vi "Measurement Logic.vi"() -> ()   [LabVIEW 2021, in "Multi-Channel Output Voltage Accuracy_PMIC.lvlib"]
uses:
  Multi-Channel Output Voltage Accuracy_PMIC.lvlib
  <instrlib>/niDCPower/nidcpower.llb/niDCPower Sense.ctl
  <instrlib>/niDCPower/nidcpower.llb/niDCPower Source Mode.ctl
  <instrlib>/niDCPower/nidcpower.llb/niDCPower Get Channel Name From String.vi
  <instrlib>/niDCPower/nidcpower.llb/niDCPower Wait For Event - Event.ctl
  Measurement Results.ctl
  <instrlib>/niDCPower/nidcpower.llb/niDCPower Configure Digital Edge Source Trigger.vi
  <instrlib>/niDCPower/nidcpower.llb/niDCPower Configure Digital Edge Measure Trigger.vi
  Measurement Configuration.ctl
  <vilib>/Plug-In SDKs/Measurements/Measure Call Context/Measure Call Context.lvclass
panel:
  out "measure call context out":refnum<class "Measure Call Context.lvclass">
  in  "measure call context in":refnum<class "Measure Call Context.lvclass">
  out "measurement results":T1
  in  "measurement configuration":T2={"Mode of operation"=enum."Perform measurement", "DUT setup time"=1.0, "Aperture time"=0.005, "Measurement time"=1.0, "Source resource name"="", "Source voltage level"=6.0, "Source current limit"=10.0, "Load resource names"=[], "Output channel alias"=[], "Load current levels"=[], "Load voltage limit ranges"=[], "Nominal output voltages"=[]} {"Measurement time" format="%.3p"}
  out "error out":errorcluster
  in  "error in":errorcluster
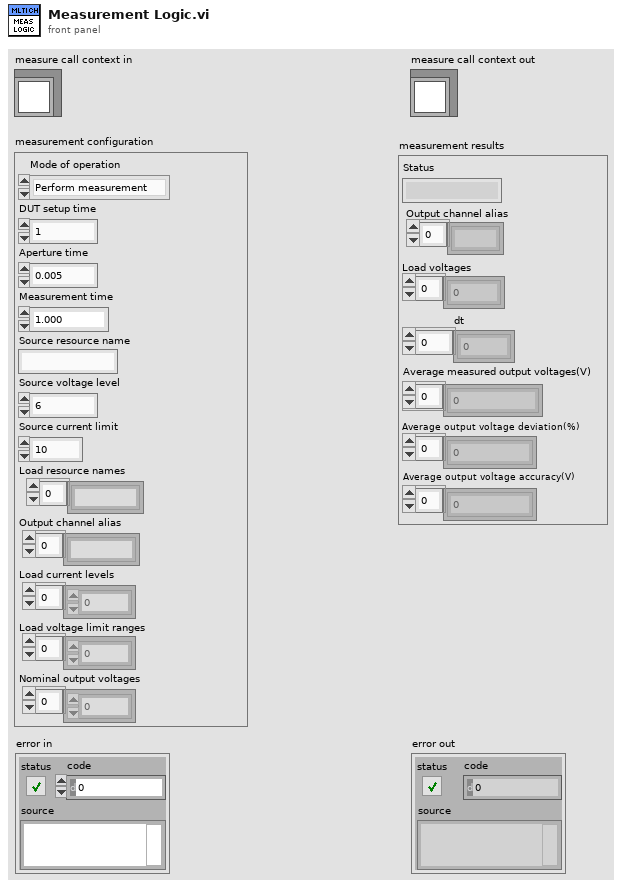
[diagram p1: front panel]
types:
  T1 = typedef "Multi-Channel Output Voltage Accuracy_PMIC.lvlib/Measurement Results.ctl" = cluster{"Status":string, "Output channel alias":string[], "Load voltages":dbl[], "dt":dbl[], "Average measured output voltages(V)":dbl[], "Average output voltage deviation(%)":dbl[], "Average output voltage accuracy(V)":dbl[]}
  T2 = typedef "Multi-Channel Output Voltage Accuracy_PMIC.lvlib/Measurement Configuration.ctl" = cluster{"Mode of operation":enum32{"Power on the DUT", "Perform measurement", "Power off the DUT"}, "DUT setup time":dbl, "Aperture time":dbl, "Measurement time":dbl, "Source resource name":string, "Source voltage level":dbl, "Source current limit":dbl, "Load resource names":string[], "Output channel alias":string[], "Load current levels":dbl[], "Load voltage limit ranges":dbl[], "Nominal output voltages":dbl[]}
  T3 = enum32{"Power on the DUT", "Perform measurement", "Power off the DUT"}
  T4 = typedef "niDCPower Wait For Event - Event.ctl" = i32
  T5 = typedef "niDCPower Source Mode.ctl" = i32
  T6 = typedef "niDCPower Sense.ctl" = i32
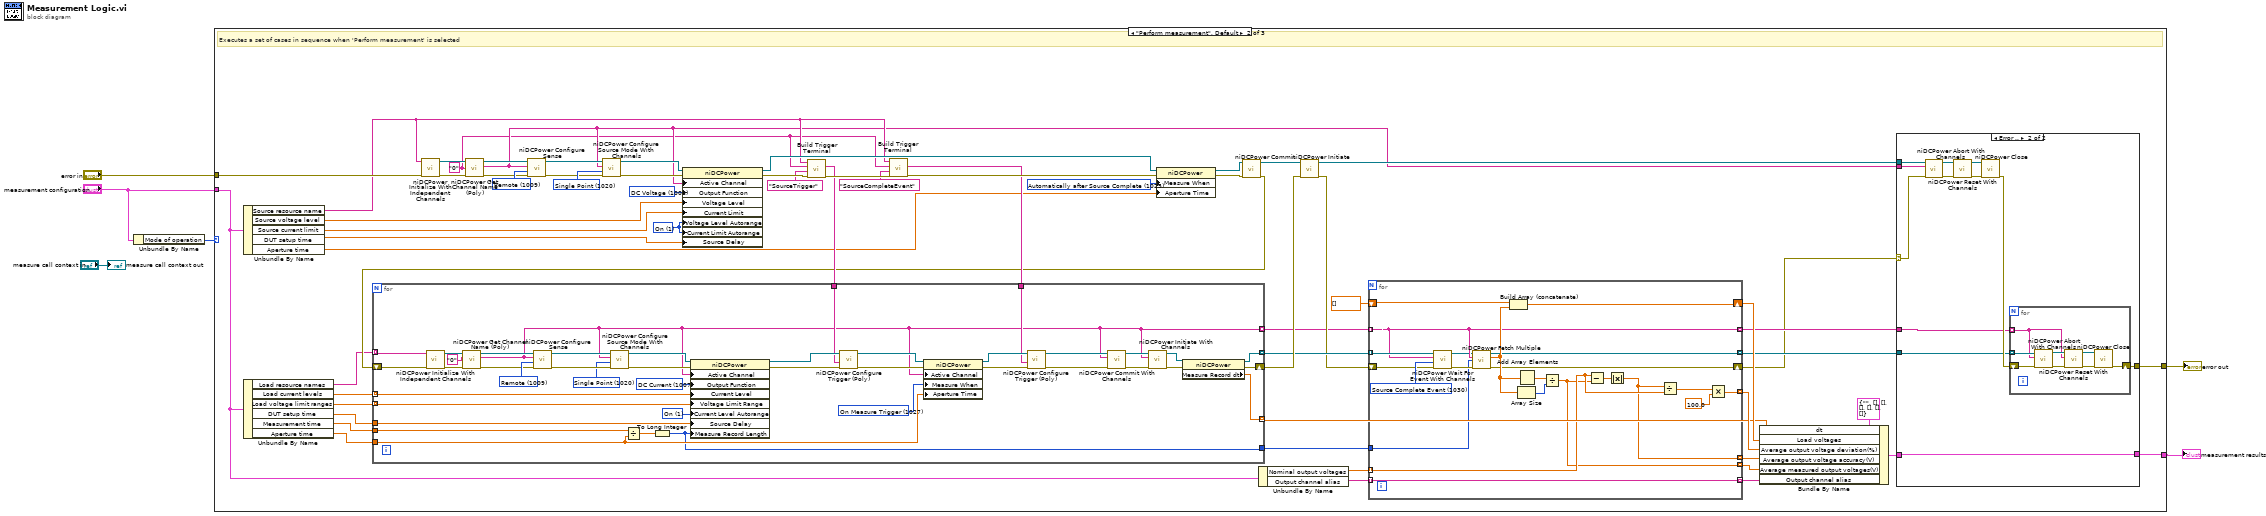
[diagram p0: block diagram]
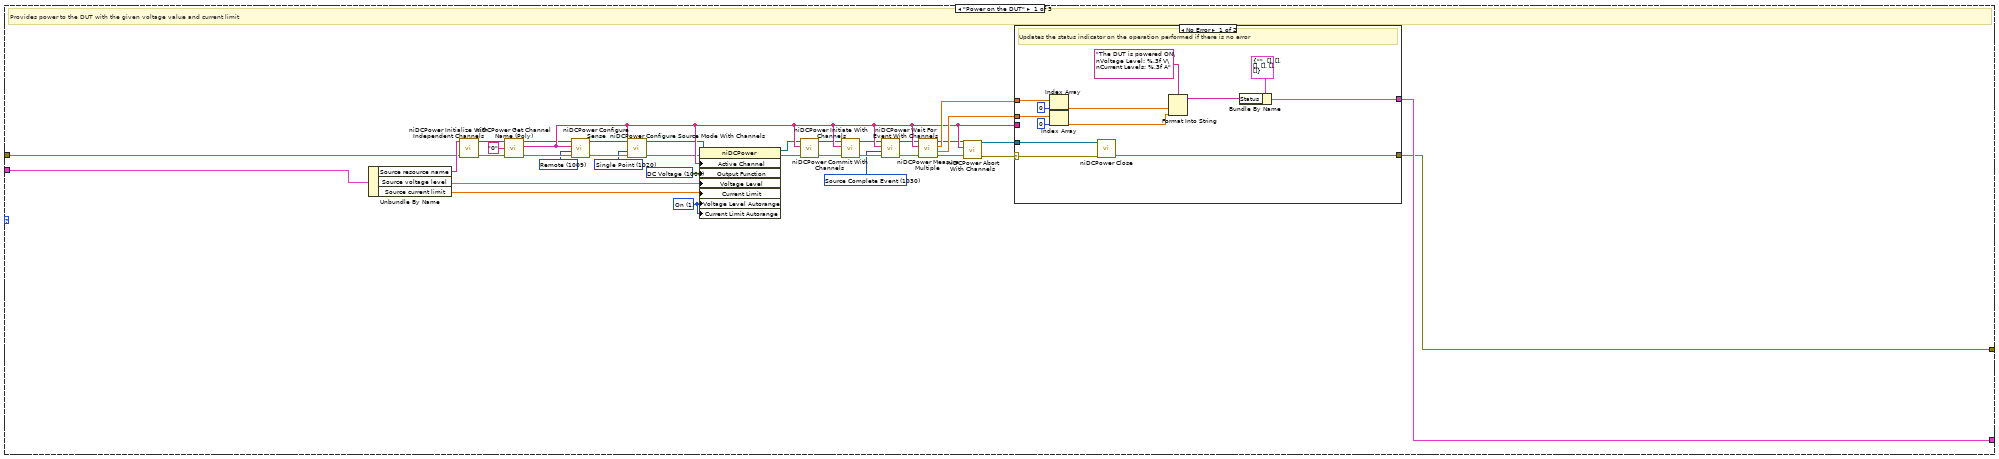
[diagram p2: hidden frame]
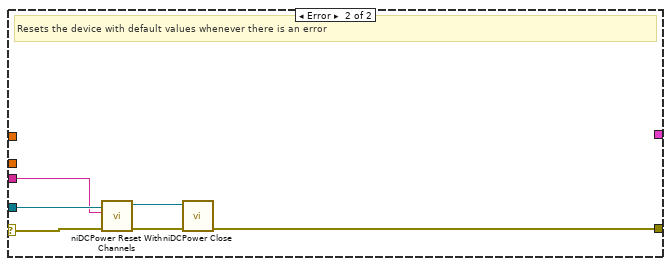
[diagram p3: hidden frame]
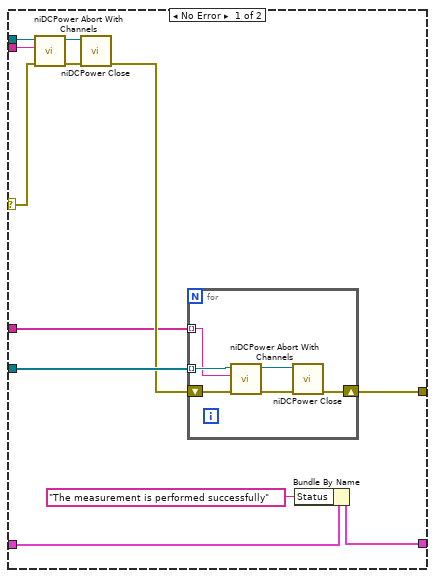
[diagram p4: hidden frame]
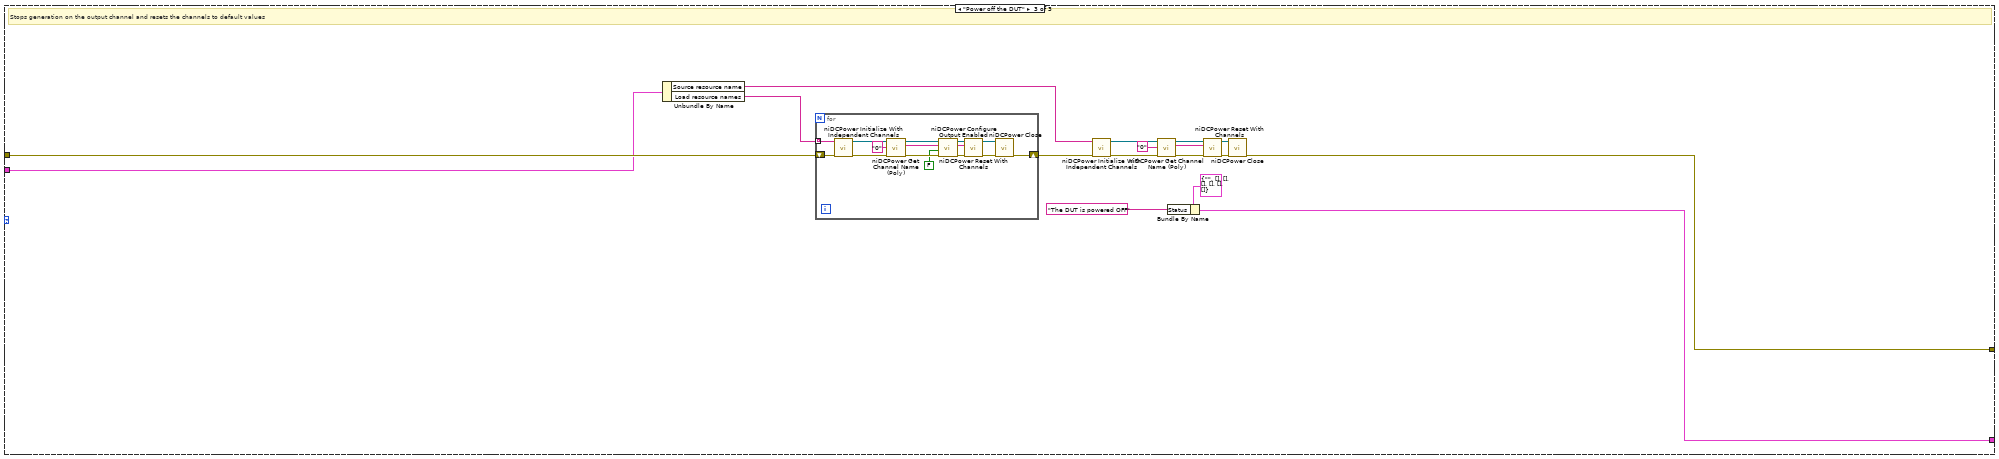
[diagram p5: hidden frame]
diagram:
  n1 = Unbundle By Name("measurement configuration") -> ("Mode of operation"=w4:T3)
  n2 = case shown="\"Perform measurement\", Default" w4 {
    tunnel: "measurement configuration" -> [w8 w89 w227]
    tunnel: "error in" -> [w10 w75 w228]
    tunnel: [w7 w74 w226] -> w2
    tunnel: [w9 w69 w224] -> w1
    frame "Power on the DUT" {
      w14 = 1 items=["Off", "On"] ("Source:DC Voltage:Voltage Level Autorange")
      w13 = T4 1030 items=["Source Complete Event"=1030, "Measure Complete Event"=1031, "Sequence Iteration Complete Event"=1032, "Sequence Engine Done Event"=1033, "Pulse Complete Event"=1051, "Ready For Pulse Trigger Event"=1052] ("event")
      w12 = T5 1020 items=["Single Point"=1020, "Sequence"=1021] ("source mode")
      w15 = 1006 items=["DC Voltage"=1006, "DC Current"=1007, "Pulse Voltage"=1049, "Pulse Current"=1050] ("Source:Output Function")
      w16 = T6 1009 items=["Local"=1008, "Remote"=1009] ("sense")
      # "Provides power to the DUT with the given voltage value and current limit"
      n3 = Unbundle By Name(w8) -> ("Source resource name"=w32:string, "Source voltage level"=w36:dbl, "Source current limit"=w31:dbl)
      n4 = call <instrlib>:"niDCPower Initialize With Independent Channels.vi"("error in (no error)"=w10, "resource name"=w32) -> ("error out"=w29:errorcluster, "instrument handle out"=w28:refnum<k15>)  [unwired: 8 in]
      n5 = call-poly <instrlib>:"niDCPower Get Channel Name (Poly).vi"("index"="0", "instrument handle"=w28) -> ("name"=w39:string, "instrument handle out"=w30:refnum<k15>)  [unwired: 7 in, 1 out]
      n6 = call <instrlib>:"niDCPower Configure Sense.vi"("error in (no error)"=w29, "sense"=w16, "channel name"=w39, "instrument handle"=w30) -> ("error out"=w22:errorcluster, "instrument handle out"=w24:refnum<k15>)  [unwired: 6 in]
      n7 = call <instrlib>:"niDCPower Configure Source Mode With Channels.vi"("error in (no error)"=w22, "source mode"=w12, "channel name"=w39, "instrument handle"=w24) -> ("error out"=w21:errorcluster, "instrument handle out"=w23:refnum<k15>)  [unwired: 6 in]
      n8 = property class="niDCPower"(reference=w23, error in=w21, "Active Channel"=w39, "Output Function"=w15, "Voltage Level"=w36, "Current Limit"=w31, "Voltage Level Autorange"=w14, "Current Limit Autorange"=w14) -> (reference out=w20:refnum<k15>, error out=w19:errorcluster)
      n9 = call <instrlib>:"niDCPower Commit With Channels.vi"("error in (no error)"=w19, "channel name"=w39, "instrument handle"=w20) -> ("error out"=w17:errorcluster, "instrument handle out"=w18:refnum<k15>)  [unwired: 7 in]
      n10 = call <instrlib>:"niDCPower Initiate With Channels.vi"("error in (no error)"=w17, "channel name"=w39, "instrument handle"=w18) -> ("error out"=w27:errorcluster, "instrument handle out"=w26:refnum<k15>)  [unwired: 7 in]
      n11 = call <instrlib>:"niDCPower Wait For Event With Channels.vi"("error in (no error)"=w27, "event"=w13, "channel name"=w39, "instrument handle"=w26) -> ("error out"=w34:errorcluster, "instrument handle out"=w25:refnum<k15>)  [unwired: 6 in]
      n12 = call <instrlib>:"niDCPower Measure Multiple.vi"("error in (no error)"=w34, "channel name"=w39, "instrument handle"=w25) -> ("error out"=w35:errorcluster, "current measurements"=w41:dbl[], "voltage measurements"=w40:dbl[], "instrument handle out"=w33:refnum<k15>)  [unwired: 5 in]
      n13 = call <instrlib>:"niDCPower Abort With Channels.vi"("error in (no error)"=w35, "channel name"=w39, "instrument handle"=w33) -> ("error out"=w37:errorcluster, "instrument handle out"=w38:refnum<k15>)  [unwired: 7 in]
      n14 = case shown="No Error" w37 {
        selector: w37 -> [w54 w58]
        tunnel: [w53 w57] -> w7
        tunnel: [w42 _] -> w9
        tunnel: w38 -> [w48 w56]
        tunnel: w39 -> [_ w55]
        tunnel: w40 -> [w47 _]
        tunnel: w41 -> [w46 _]
        frame No Error {
          # "Updates the status indicator on the operation performed if there is no error"
          n15 = Index Array(array=w47, index=0) -> (element=w45:dbl)
          n16 = Index Array(array=w46, index=0) -> (element=w44:dbl)
          n17 = call <instrlib>:"niDCPower Close.vi"("error in (no error)"=w54, "instrument handle"=w48) -> ("error out"=w53:errorcluster)  [unwired: 9 out]
          n18 = Format Into String(format string="The DUT is powered ON\nVoltage Level: %.3f V\nCurrent Levels: %.3f A" ("message"), w45, w44) -> (resulting string=w51:string)  [unwired: 2 in, 1 out]
          n19 = Bundle By Name(cluster=T1 {"Status"="", "Output channel alias"=[], "Load voltages"=[], "dt"=[], "Average measured output voltages(V)"=[], "Average output voltage deviation(%)"=[], "Average output voltage accuracy(V)"=[]} ("measurement results"), "Status"=w51) -> (w42:T1)
        }
        frame Error {
          # "Resets the device with default values whenever there is an error"
          n20 = call <instrlib>:"niDCPower Reset With Channels.vi"("error in (no error)"=w58, "channel name"=w55, "instrument handle"=w56) -> ("error out"=w60:errorcluster, "instrument handle out"=w59:refnum<k15>)  [unwired: 7 in]
          n21 = call <instrlib>:"niDCPower Close.vi"("error in (no error)"=w60, "instrument handle"=w59) -> ("error out"=w57:errorcluster)  [unwired: 9 out]
        }
      }
    }
    frame "Perform measurement", Default {
      w111 = 1025 items=["Automatically after Source Complete"=1025, "On Demand"=1026, "On Measure Trigger"=1027] ("Measurement:Advanced:Measure When")
      w63 = "0" ("index")
      w115 = 1 items=["Off", "On"] ("Source:DC Voltage:Voltage Level Autorange")
      w122 = T5 1020 items=["Single Point"=1020, "Sequence"=1021] ("source mode")
      w118 = 1006 items=["DC Voltage"=1006, "DC Current"=1007, "Pulse Voltage"=1049, "Pulse Current"=1050] ("Source:Output Function")
      w116 = T6 1009 items=["Local"=1008, "Remote"=1009] ("sense")
      # "Executes a set of cases in sequence when 'Perform measurement' is selected"
      n22 = Unbundle By Name(w89) -> ("Source resource name"=w73:string, "Source voltage level"=w107:dbl, "Source current limit"=w106:dbl, "DUT setup time"=w105:dbl, "Aperture time"=w76:dbl)
      n23 = Unbundle By Name(w89) -> ("Load resource names"=w99:string[], "Load current levels"=w98:dbl[], "Load voltage limit ranges"=w97:dbl[], "DUT setup time"=w96:dbl, "Measurement time"=w90:dbl, "Aperture time"=w91:dbl)
      n24 = call <instrlib>:"niDCPower Initialize With Independent Channels.vi"("error in (no error)"=w75, "resource name"=w73) -> ("error out"=w62:errorcluster, "instrument handle out"=w117:refnum<k15>)  [unwired: 8 in]
      n25 = call-poly <instrlib>:"niDCPower Get Channel Name (Poly).vi"("error in (no error)"=w62, "index"=w63, "instrument handle"=w117) -> ("error out"=w61:errorcluster, "name"=w64:string, "instrument handle out"=w114:refnum<k15>)  [unwired: 6 in]
      n26 = call <instrlib>:"niDCPower Configure Sense.vi"("error in (no error)"=w61, "sense"=w116, "channel name"=w64, "instrument handle"=w114) -> ("error out"=w120:errorcluster, "instrument handle out"=w119:refnum<k15>)  [unwired: 6 in]
      n27 = call <instrlib>:"niDCPower Configure Source Mode With Channels.vi"("error in (no error)"=w120, "source mode"=w122, "channel name"=w64, "instrument handle"=w119) -> ("error out"=w121:errorcluster, "instrument handle out"=w104:refnum<k15>)  [unwired: 6 in]
      n28 = property class="niDCPower"(reference=w104, error in=w121, "Active Channel"=w64, "Output Function"=w118, "Voltage Level"=w107, "Current Limit"=w106, "Voltage Level Autorange"=w115, "Current Limit Autorange"=w115, "Source Delay"=w105) -> (reference out=w103:refnum<k15>, error out=w110:errorcluster)
      n29 = call "Build Trigger Terminal.vi"("error in (no error)"=w110, "Trigger/Event Name"="SourceTrigger", "Channel Name"=w63, "Resource Name"=w73) -> ("error out"=w109:errorcluster, "Terminal Name"=w102:string)  [unwired: 6 in]
      n30 = call "Build Trigger Terminal.vi"("error in (no error)"=w109, "Trigger/Event Name"="SourceCompleteEvent", "Channel Name"=w63, "Resource Name"=w73) -> ("error out"=w108:errorcluster, "Terminal Name"=w101:string)  [unwired: 6 in]
      n31 = property class="niDCPower"(reference=w103, error in=w108, "Measure When"=w111, "Aperture Time"=w76) -> (reference out=w113:refnum<k15>, error out=w112:errorcluster)
      n32 = call <instrlib>:"niDCPower Commit.vi"("error in (no error)"=w112, "instrument handle"=w113) -> ("error out"=w100:errorcluster, "instrument handle out"=w95:refnum<k15>)  [unwired: 8 out]
      n33 = for {
        tunnel: w91 -> [w192]
        tunnel: [w187] -> w93 mode=indexing
        tunnel: w102 -> [w200]
        tunnel: w101 -> [w199]
        tunnel: w96 -> [w195]
        shift-right: [w189] -> w94
        shift-left: w100 -> [w201]
        tunnel: w99 -> [w198] mode=indexing
        tunnel: w98 -> [w197] mode=indexing
        tunnel: w97 -> [w196] mode=indexing
        tunnel: w90 -> [w194]
        tunnel: [w191] -> w72
        tunnel: [w185] -> w78 mode=indexing
        tunnel: [w186] -> w67 mode=indexing
        w206 = 1027 items=["Automatically after Source Complete"=1025, "On Demand"=1026, "On Measure Trigger"=1027] ("Measurement:Advanced:Measure When")
        w211 = 1 items=["Off", "On"] ("Source:DC Current:Current Level Autorange")
        w212 = 1007 items=["DC Voltage"=1006, "DC Current"=1007, "Pulse Voltage"=1049, "Pulse Current"=1050] ("Source:Output Function")
        w215 = T5 1020 items=["Single Point"=1020, "Sequence"=1021] ("source mode")
        w221 = T6 1009 items=["Local"=1008, "Remote"=1009] ("sense")
        n34 = call <instrlib>:"niDCPower Initialize With Independent Channels.vi"("error in (no error)"=w201, "resource name"=w198) -> ("error out"=w184:errorcluster, "instrument handle out"=w220:refnum<k15>)  [unwired: 8 in]
        n35 = call-poly <instrlib>:"niDCPower Get Channel Name (Poly).vi"("error in (no error)"=w184, "index"="0", "instrument handle"=w220) -> ("error out"=w183:errorcluster, "name"=w185:string, "instrument handle out"=w222:refnum<k15>)  [unwired: 6 in]
        n36 = call <instrlib>:"niDCPower Configure Sense.vi"("error in (no error)"=w183, "sense"=w221, "channel name"=w185, "instrument handle"=w222) -> ("error out"=w217:errorcluster, "instrument handle out"=w219:refnum<k15>)  [unwired: 6 in]
        n37 = call <instrlib>:"niDCPower Configure Source Mode With Channels.vi"("error in (no error)"=w217, "source mode"=w215, "channel name"=w185, "instrument handle"=w219) -> ("error out"=w216:errorcluster, "instrument handle out"=w218:refnum<k15>)  [unwired: 6 in]
        n38 = Divide(x=w194, y=w192) -> (x/y=w193:dbl)
        n39 = To Long Integer(number=w193) -> (32bit integer=w191:i32)
        n40 = property class="niDCPower"(reference=w218, error in=w216, "Active Channel"=w185, "Output Function"=w212, "Current Level"=w197, "Voltage Limit Range"=w196, "Current Level Autorange"=w211, "Source Delay"=w195, "Measure Record Length"=w191) -> (reference out=w202:refnum<k15>, error out=w205:errorcluster)
        n41 = call-poly <instrlib>:"niDCPower Configure Trigger (Poly).vi"("error in (no error)"=w205, "input terminal"=w200, "instrument handle"=w202) -> ("error out"=w209:errorcluster, "instrument handle out"=w210:refnum<k15>)  [unwired: 1 in, 6 out]
        n42 = property class="niDCPower"(reference=w210, error in=w209, "Active Channel"=w185, "Measure When"=w206, "Aperture Time"=w192) -> (reference out=w207:refnum<k15>, error out=w208:errorcluster)
        n43 = call-poly <instrlib>:"niDCPower Configure Trigger (Poly).vi"("error in (no error)"=w208, "input terminal"=w199, "instrument handle"=w207) -> ("error out"=w204:errorcluster, "instrument handle out"=w203:refnum<k15>)  [unwired: 1 in, 6 out]
        n44 = call <instrlib>:"niDCPower Commit With Channels.vi"("error in (no error)"=w204, "channel name"=w185, "instrument handle"=w203) -> ("error out"=w214:errorcluster, "instrument handle out"=w213:refnum<k15>)  [unwired: 7 in]
        n45 = call <instrlib>:"niDCPower Initiate With Channels.vi"("error in (no error)"=w214, "channel name"=w185, "instrument handle"=w213) -> ("error out"=w190:errorcluster, "instrument handle out"=w188:refnum<k15>)  [unwired: 7 in]
        n46 = property class="niDCPower"(reference=w188, error in=w190) -> (reference out=w187:refnum<k15>, error out=w189:errorcluster, "Measure Record dt"=w186:dbl)
      }
      n47 = Unbundle By Name(w89) -> ("Nominal output voltages"=w88:dbl[], "Output channel alias"=w87:string[])
      n48 = call <instrlib>:"niDCPower Initiate.vi"("error in (no error)"=w94, "instrument handle"=w95) -> ("error out"=w92:errorcluster, "instrument handle out"=w79:refnum<k15>)  [unwired: 8 out]
      n49 = for {
        shift-right: [w163] -> w68
        shift-left: w92 -> [w181]
        tunnel: [w165] -> w80 mode=indexing
        tunnel: w93 -> [w180] mode=indexing
        tunnel: w88 -> [w174] mode=indexing
        tunnel: [w161] -> w71 mode=indexing
        tunnel: [w173] -> w83 mode=indexing
        tunnel: [w172] -> w84 mode=indexing
        tunnel: [w171] -> w85 mode=indexing
        tunnel: w87 -> [w171] mode=indexing
        shift-right: [w168] -> w81
        shift-left: dbl[] [] -> [w170]
        tunnel: w78 -> [w167] mode=indexing
        tunnel: [w167] -> w77 mode=indexing
        tunnel: w72 -> [w162]
        w182 = T4 1030 items=["Source Complete Event"=1030, "Measure Complete Event"=1031, "Sequence Iteration Complete Event"=1032, "Sequence Engine Done Event"=1033, "Pulse Complete Event"=1051, "Ready For Pulse Trigger Event"=1052] ("event")
        n50 = call <instrlib>:"niDCPower Wait For Event With Channels.vi"("error in (no error)"=w181, "event"=w182, "channel name"=w167, "instrument handle"=w180) -> ("error out"=w164:errorcluster, "instrument handle out"=w166:refnum<k15>)  [unwired: 6 in]
        n51 = call <instrlib>:"niDCPower Fetch Multiple.vi"("instrument handle"=w166, "channel name"=w167, "count (1)"=w162, "error in (no error)"=w164) -> ("instrument handle out"=w165:refnum<k15>, "voltage measurements"=w169:dbl[], "error out"=w163:errorcluster)  [unwired: 6 in, 3 out]
        n52 = Build Array (concatenate)(w170, w169) -> (w168:dbl[])
        n53 = Add Array Elements(numeric array=w169) -> (sum=w176:dbl)
        n54 = Array Size(array=w169) -> (size(s)=w175:i32)
        n55 = Divide(x=w176, y=w175) -> (x/y=w172:dbl)
        n56 = Subtract(x=w174, y=w172) -> (x-y=w177:dbl)
        n57 = Absolute Value(x=w177) -> (abs(x)=w161:dbl)
        n58 = Divide(x=w161, y=w174) -> (x/y=w179:dbl)
        n59 = Multiply(x=w179, y=100.0) -> (x*y=w173:dbl)
      }
      n60 = Bundle By Name(cluster=T1 {"Status"="", "Output channel alias"=[], "Load voltages"=[], "dt"=[], "Average measured output voltages(V)"=[], "Average output voltage deviation(%)"=[], "Average output voltage accuracy(V)"=[]} ("measurement results"), "dt"=w67, "Load voltages"=w81, "Average output voltage deviation(%)"=w83, "Average output voltage accuracy(V)"=w71, "Average measured output voltages(V)"=w84, "Output channel alias"=w85) -> (w70:T1)
      n61 = case shown="Error .." w68 {
        selector: w68 -> [w123 w143]
        tunnel: w80 -> [w134 w151]
        tunnel: w79 -> [w130 w149]
        tunnel: w77 -> [w129 w150]
        tunnel: [w128 w142] -> w74
        tunnel: w64 -> [w127 w148]
        tunnel: w70 -> [w125 w141]
        tunnel: [w126 w141] -> w69
        frame No Error {
          n62 = call <instrlib>:"niDCPower Abort With Channels.vi"("error in (no error)"=w123, "channel name"=w127, "instrument handle"=w130) -> ("error out"=w133:errorcluster, "instrument handle out"=w132:refnum<k15>)  [unwired: 7 in]
          n63 = call <instrlib>:"niDCPower Close.vi"("error in (no error)"=w133, "instrument handle"=w132) -> ("error out"=w131:errorcluster)  [unwired: 9 out]
          n64 = for {
            shift-right: [w139] -> w128
            shift-left: w131 -> [w140]
            tunnel: w134 -> [w136] mode=indexing
            tunnel: w129 -> [w135] mode=indexing
            n65 = call <instrlib>:"niDCPower Abort With Channels.vi"("error in (no error)"=w140, "channel name"=w135, "instrument handle"=w136) -> ("error out"=w138:errorcluster, "instrument handle out"=w137:refnum<k15>)  [unwired: 7 in]
            n66 = call <instrlib>:"niDCPower Close.vi"("error in (no error)"=w138, "instrument handle"=w137) -> ("error out"=w139:errorcluster)  [unwired: 9 out]
          }
          n67 = Bundle By Name(cluster=w125, "Status"="The measurement is performed successfully" ("message")) -> (w126:T1)
        }
        frame Error {
          n68 = call <instrlib>:"niDCPower Abort With Channels.vi"("error in (no error)"=w143, "channel name"=w148, "instrument handle"=w149) -> ("error out"=w145:errorcluster, "instrument handle out"=w147:refnum<k15>)  [unwired: 7 in]
          n69 = call <instrlib>:"niDCPower Reset With Channels.vi"("error in (no error)"=w145, "instrument handle"=w147) -> ("error out"=w144:errorcluster, "instrument handle out"=w146:refnum<k15>)  [unwired: 8 in]
          n70 = call <instrlib>:"niDCPower Close.vi"("error in (no error)"=w144, "instrument handle"=w146) -> ("error out"=w152:errorcluster)  [unwired: 9 out]
          n71 = for {
            shift-right: [w159] -> w142
            shift-left: w152 -> [w160]
            tunnel: w151 -> [w158] mode=indexing
            tunnel: w150 -> [w153] mode=indexing
            n72 = call <instrlib>:"niDCPower Abort With Channels.vi"("error in (no error)"=w160, "channel name"=w153, "instrument handle"=w158) -> ("error out"=w157:errorcluster, "instrument handle out"=w155:refnum<k15>)  [unwired: 7 in]
            n73 = call <instrlib>:"niDCPower Reset With Channels.vi"("error in (no error)"=w157, "channel name"=w153, "instrument handle"=w155) -> ("error out"=w156:errorcluster, "instrument handle out"=w154:refnum<k15>)  [unwired: 7 in]
            n74 = call <instrlib>:"niDCPower Close.vi"("error in (no error)"=w156, "instrument handle"=w154) -> ("error out"=w159:errorcluster)  [unwired: 9 out]
          }
        }
      }
    }
    frame "Power off the DUT" {
      # "Stops generation on the output channel and resets the channels to default values"
      n75 = Unbundle By Name(w227) -> ("Source resource name"=w239:string, "Load resource names"=w237:string[])
      n76 = for {
        tunnel: w237 -> [w253] mode=indexing
        shift-right: [w251] -> w234
        shift-left: w228 -> [w241]
        n77 = call <instrlib>:"niDCPower Initialize With Independent Channels.vi"("error in (no error)"=w241, "resource name"=w253) -> ("error out"=w252:errorcluster, "instrument handle out"=w254:refnum<k15>)  [unwired: 8 in]
        n78 = call-poly <instrlib>:"niDCPower Get Channel Name (Poly).vi"("error in (no error)"=w252, "index"="0", "instrument handle"=w254) -> ("error out"=w248:errorcluster, "name"=w250:string, "instrument handle out"=w249:refnum<k15>)  [unwired: 6 in]
        n79 = call <instrlib>:"niDCPower Configure Output Enabled.vi"("error in (no error)"=w248, "output enabled"=FALSE, "channel name"=w250, "instrument handle"=w249) -> ("error out"=w244:errorcluster, "instrument handle out"=w245:refnum<k15>)  [unwired: 6 in]
        n80 = call <instrlib>:"niDCPower Reset With Channels.vi"("error in (no error)"=w244, "channel name"=w250, "instrument handle"=w245) -> ("error out"=w247:errorcluster, "instrument handle out"=w246:refnum<k15>)  [unwired: 7 in]
        n81 = call <instrlib>:"niDCPower Close.vi"("error in (no error)"=w247, "instrument handle"=w246) -> ("error out"=w251:errorcluster)  [unwired: 9 out]
      }
      n82 = call <instrlib>:"niDCPower Initialize With Independent Channels.vi"("error in (no error)"=w234, "resource name"=w239) -> ("error out"=w238:errorcluster, "instrument handle out"=w240:refnum<k15>)  [unwired: 8 in]
      n83 = call-poly <instrlib>:"niDCPower Get Channel Name (Poly).vi"("error in (no error)"=w238, "index"="0", "instrument handle"=w240) -> ("error out"=w235:errorcluster, "name"=w236:string, "instrument handle out"=w233:refnum<k15>)  [unwired: 6 in]
      n84 = Bundle By Name(cluster=T1 {"Status"="", "Output channel alias"=[], "Load voltages"=[], "dt"=[], "Average measured output voltages(V)"=[], "Average output voltage deviation(%)"=[], "Average output voltage accuracy(V)"=[]} ("measurement results"), "Status"="The DUT is powered OFF" ("Measurement Results.Status")) -> (w224:T1)
      n85 = call <instrlib>:"niDCPower Reset With Channels.vi"("error in (no error)"=w235, "channel name"=w236, "instrument handle"=w233) -> ("error out"=w231:errorcluster, "instrument handle out"=w232:refnum<k15>)  [unwired: 7 in]
      n86 = call <instrlib>:"niDCPower Close.vi"("error in (no error)"=w231, "instrument handle"=w232) -> ("error out"=w226:errorcluster)  [unwired: 9 out]
    }
  }
  "error out" <- w2
  "measurement results" <- w1
  "measure call context out" <- "measure call context in"
